vi "TL_ALL_on.vi"(10 "Settings":T2={"Module"=enum."On Line LD", "OnLineTEC"=19.636, "OnLineLD"=0.150051534, "OffLineTEC"=18.68, "OffLineLD"=0.150183529, "EtalonTEC"=28.1496544, "TSOA-TEC"=20.0007572} {"OffLineLD" min=0.0 max=0.17 step=0.001 format="%.3p"; "OnLineLD" min=0.0 max=0.17 step=0.001 format="%.3p"; "TSOA-TEC" format="%.2g"; "EtalonTEC" format="%.2g"; "OffLineTEC" min=16.0 max=28.0 step=0.1 format="%.3g"; "OnLineTEC" min=16.0 max=28.0 step=0.1 format="%.3g"}, 11 "Device In":refnum<visa-resource-name>="ThorLabs") -> ()   [LabVIEW 2012]
panel:
  out "Readings":T1={"OnLineTEC"=19.6625309, "OnLineLD"=0.150554702, "OffLineTEC"=18.6780949, "OffLineLD"=0.149925783, "EtalonTEC"=28.1907768, "TSOA-TEC"=21.1046085, "Pro8000"=TRUE, "OnLine TEC"=TRUE, "OnLine LD"=TRUE, "OffLine TEC"=TRUE, "OffLine LD"=TRUE, "Etalon TEC"=TRUE, "TSOA TEC"=TRUE} {"OffLineLD" format="%.3p"; "OnLineLD" format="%.3p"; "TSOA-TEC" format="%.3g"; "EtalonTEC" format="%.3g"; "OffLineTEC" format="%.3g"; "OnLineTEC" format="%.3g"}
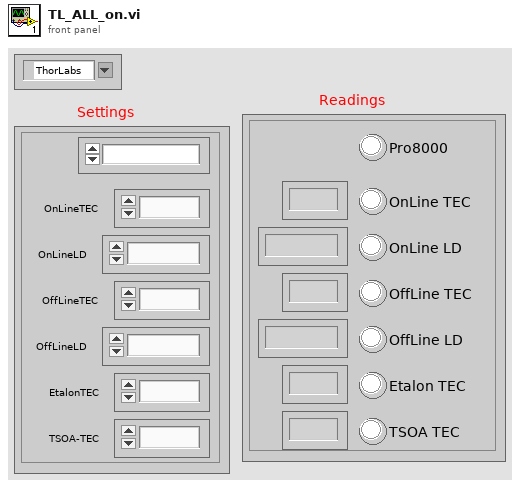
[diagram p1: front panel]
types:
  T1 = cluster{"OnLineTEC":dbl, "OnLineLD":dbl, "OffLineTEC":dbl, "OffLineLD":dbl, "EtalonTEC":dbl, "TSOA-TEC":dbl, "Pro8000":bool, "OnLine TEC":bool, "OnLine LD":bool, "OffLine TEC":bool, "OffLine LD":bool, "Etalon TEC":bool, "TSOA TEC":bool}
  T2 = cluster{"Module":enum16{"On Line TEC", "On Line LD", "Off Line TEC", "Off Line LD", "Etalon TEC", "TSOA TEC"}, "OnLineTEC":dbl, "OnLineLD":dbl, "OffLineTEC":dbl, "OffLineLD":dbl, "EtalonTEC":dbl, "TSOA-TEC":dbl}
  T3 = enum16{"Open_TL", "Close_TL", "Verify_ID", "TEC_Sensor", "SET", "READ", "ON", "OFF", "Set_Limits", "Read_Limits", "Enable_Status", "Read_Status"}
  T4 = enum16{"On Line TEC", "On Line LD", "Off Line TEC", "Off Line LD", "Etalon TEC", "TSOA TEC"}
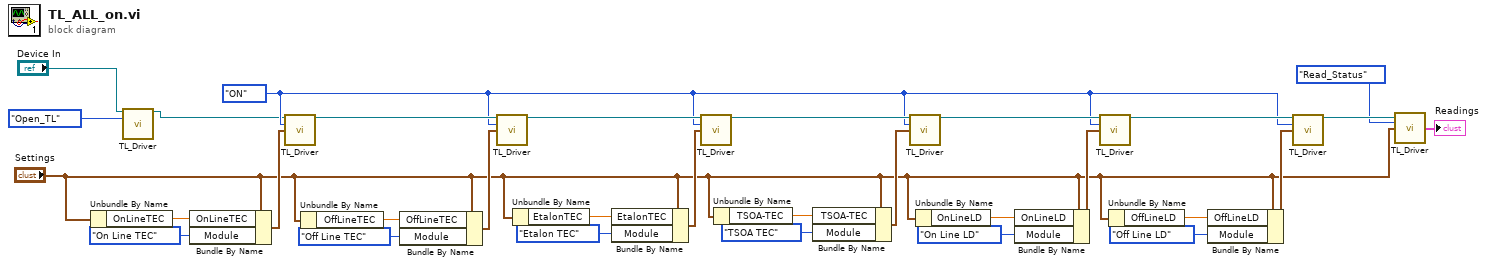
[diagram p0: block diagram]
diagram:
  w9 = T3."ON" ("Commands")
  n1 = Unbundle By Name("Settings") -> ("OnLineTEC"=w27:dbl)
  n2 = call "TL_Driver.vi"("Device In"="Device In", "Commands"=T3."Open_TL") -> ("Device Out"=w3:refnum<visa-resource-name>)  [unwired: 10 in, 3 out]
  n3 = Bundle By Name(cluster="Settings", "OnLineTEC"=w27, "Module"=T4."On Line TEC") -> (w25:T2)
  n4 = call "TL_Driver.vi"("Device In"=w3, "Commands"=w9, "Settings"=w25) -> ("Device Out"=w31:refnum<visa-resource-name>)  [unwired: 9 in, 3 out]
  n5 = Unbundle By Name("Settings") -> ("OffLineTEC"=w24:dbl)
  n6 = Bundle By Name(cluster="Settings", "OffLineTEC"=w24, "Module"=T4."Off Line TEC") -> (w22:T2)
  n7 = call "TL_Driver.vi"("Device In"=w31, "Commands"=w9, "Settings"=w22) -> ("Device Out"=w30:refnum<visa-resource-name>)  [unwired: 9 in, 3 out]
  n8 = Unbundle By Name("Settings") -> ("EtalonTEC"=w21:dbl)
  n9 = Bundle By Name(cluster="Settings", "EtalonTEC"=w21, "Module"=T4."Etalon TEC") -> (w19:T2)
  n10 = call "TL_Driver.vi"("Device In"=w30, "Commands"=w9, "Settings"=w19) -> ("Device Out"=w29:refnum<visa-resource-name>)  [unwired: 9 in, 3 out]
  n11 = Unbundle By Name("Settings") -> ("TSOA-TEC"=w18:dbl)
  n12 = Bundle By Name(cluster="Settings", "TSOA-TEC"=w18, "Module"=T4."TSOA TEC") -> (w16:T2)
  n13 = call "TL_Driver.vi"("Device In"=w29, "Commands"=w9, "Settings"=w16) -> ("Device Out"=w28:refnum<visa-resource-name>)  [unwired: 9 in, 3 out]
  n14 = Unbundle By Name("Settings") -> ("OnLineLD"=w15:dbl)
  n15 = Bundle By Name(cluster="Settings", "OnLineLD"=w15, "Module"=T4."On Line LD") -> (w13:T2)
  n16 = call "TL_Driver.vi"("Device In"=w28, "Commands"=w9, "Settings"=w13) -> ("Device Out"=w10:refnum<visa-resource-name>)  [unwired: 9 in, 3 out]
  n17 = Unbundle By Name("Settings") -> ("OffLineLD"=w12:dbl)
  n18 = Bundle By Name(cluster="Settings", "OffLineLD"=w12, "Module"=T4."Off Line LD") -> (w8:T2)
  n19 = call "TL_Driver.vi"("Device In"=w10, "Commands"=w9, "Settings"=w8) -> ("Device Out"=w7:refnum<visa-resource-name>)  [unwired: 9 in, 3 out]
  n20 = call "TL_Driver.vi"("Device In"=w7, "Commands"=T3."Read_Status", "Settings"="Settings") -> ("Readings"=→"Readings":T1)  [unwired: 9 in, 3 out]
